vi "Send Email.vi"(4 "Body":string, 5 "Attachments":path[](array[path]), 6 "Subject":string, 7 "Email Address":string, 8 "error in (no error)":errorcluster, 9 "Email Password":string, 10 "Email Username":string, 11 "SMTP Server":string) -> (0 "error out":errorcluster)   [LabVIEW 2013]
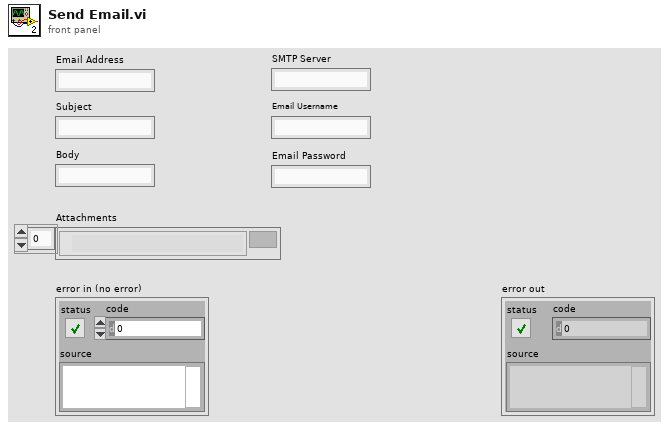
[diagram p1: front panel]
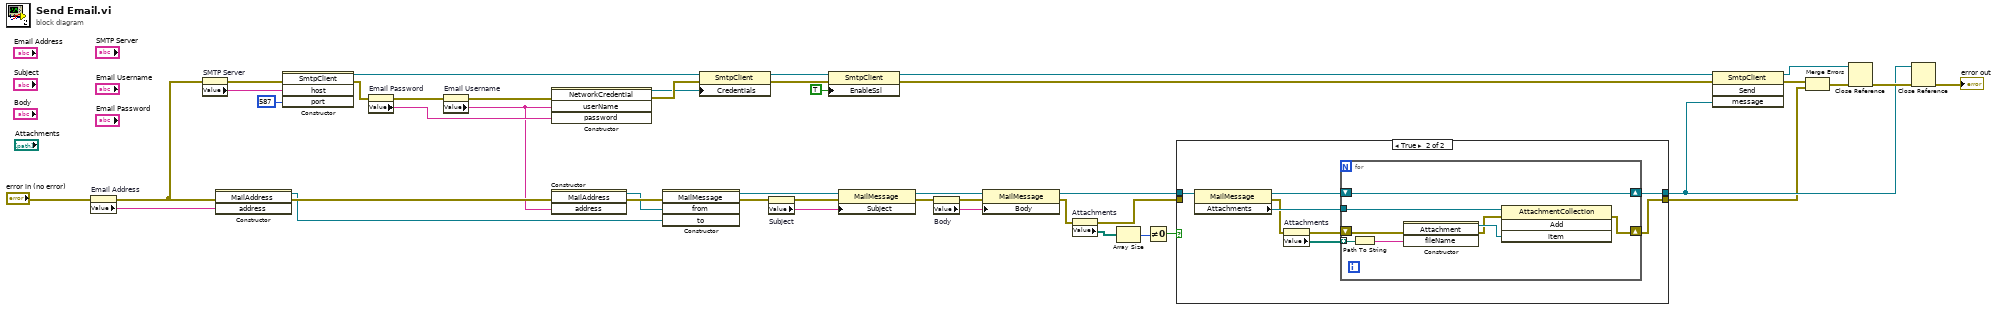
[diagram p0: block diagram]
diagram:
  n1 = property on="Email Address" class="Str"(error in="error in (no error)") -> (error out=w2:errorcluster, "Value"=w1:string)  [unwired: 1 in, 1 out]
  n2 = property on="SMTP Server" class="Str"(error in=w2) -> (error out=w21:errorcluster, "Value"=w20:string)  [unwired: 1 in, 1 out]
  n3 = constructor class="MailAddress"(error in=w2, "address"=w1) -> (reference out=w35:refnum<k24>, error out=w38:errorcluster)  [unwired: 2 in, 2 out]
  n4 = constructor class="SmtpClient"(error in=w21, "host"=w20, "port"=587) -> (reference out=w39:refnum<k24>, error out=w19:errorcluster)  [unwired: 2 in, 3 out]
  n5 = property on="Email Password" class="Str"(error in=w19) -> (error out=w43:errorcluster, "Value"=w18:string)  [unwired: 1 in, 1 out]
  n6 = property on="Email Username" class="Str"(error in=w43) -> (error out=w16:errorcluster, "Value"=w17:string)  [unwired: 1 in, 1 out]
  n7 = constructor class="NetworkCredential"(error in=w16, "userName"=w17, "password"=w18) -> (reference out=w40:refnum<k24>, error out=w41:errorcluster)  [unwired: 2 in, 3 out]
  n8 = constructor class="MailAddress"(error in=w38, "address"=w17) -> (reference out=w36:refnum<k24>, error out=w37:errorcluster)  [unwired: 2 in, 2 out]
  n9 = constructor class="MailMessage"(error in=w37, "from"=w36, "to"=w35) -> (reference out=w34:refnum<k24>, error out=w15:errorcluster)  [unwired: 2 in, 3 out]
  n10 = property class="SmtpClient"(reference=w39, error in=w41, "Credentials"=w40) -> (reference out=w31:refnum<k24>, error out=w32:errorcluster)
  n11 = property on="Subject" class="Str"(error in=w15) -> (error out=w14:errorcluster, "Value"=w13:string)  [unwired: 1 in, 1 out]
  n12 = property class="SmtpClient"(reference=w31, error in=w32, "EnableSsl"=TRUE) -> (reference out=w28:refnum<k24>, error out=w29:errorcluster)
  n13 = property class="MailMessage"(reference=w34, error in=w14, "Subject"=w13) -> (reference out=w33:refnum<k24>, error out=w12:errorcluster)
  n14 = property on="Body" class="Str"(error in=w12) -> (error out=w11:errorcluster, "Value"=w10:string)  [unwired: 1 in, 1 out]
  n15 = property class="MailMessage"(reference=w33, error in=w11, "Body"=w10) -> (reference out=w23:refnum<k24>, error out=w4:errorcluster)
  n16 = property on="Attachments" class="Arr (strict)"(error in=w4) -> (error out=w3:errorcluster, "Value"=w7:path[])  [unwired: 1 in, 1 out]
  n17 = Array Size(array=w7) -> (size(s)=w6:i32)
  n18 = Not Equal To 0?(x=w6) -> (x != 0?=w5:bool)
  n19 = case shown="True" w5 {
    tunnel: w3 -> [w46 _]
    tunnel: [w46 w47] -> w8
    tunnel: w23 -> [w45 w54]
    tunnel: [w45 w48] -> w22
    frame False {
    }
    frame True {
      n20 = property class="MailMessage"(reference=w54) -> (reference out=w51:refnum<k24>, error out=w52:errorcluster, "Attachments"=w53:refnum<k24>)  [unwired: 1 in]
      n21 = property on="Attachments" class="Arr (strict)"(error in=w52) -> (error out=w49:errorcluster, "Value"=w50:path[])  [unwired: 1 in, 1 out]
      n22 = for {
        tunnel: w53 -> [w62]
        shift-right: [w61] -> w48
        shift-left: w51 -> [w61]
        tunnel: w50 -> [w60] mode=indexing
        shift-right: [w55] -> w47
        shift-left: w49 -> [w58]
        n23 = Path To String(path=w60) -> (string=w59:string)
        n24 = constructor class="Attachment"(error in=w58, "fileName"=w59) -> (reference out=w57:refnum<k24>, error out=w56:errorcluster)  [unwired: 2 in, 2 out]
        n25 = invoke class="AttachmentCollection" method="Add"(reference=w62, error in=w56, "item"=w57) -> (error out=w55:errorcluster)  [unwired: 1 in, 3 out]
      }
    }
  }
  n26 = invoke class="SmtpClient" method="Send"(reference=w28, error in=w29, "message"=w22) -> (reference out=w25:refnum<k24>, error out=w27:errorcluster)  [unwired: 1 in, 2 out]
  n27 = Merge Errors(w27, w8) -> (w26:errorcluster)
  n28 = Close Reference(reference=w25, error in (no error)=w26) -> (error out=w24:errorcluster)
  n29 = Close Reference(reference=w22, error in (no error)=w24) -> (error out=→"error out":errorcluster)
